vi "Choreo_Util_ConvertTrajectoryToRelative.vi"(11 "ChoreoTrajectory":T1) -> (3 "Flipped Trajectory":T1)   [LabVIEW 2019]
doc: "trajectory, mirrored across the field midline.\n\nInputs: \n - ChoreoTrajectory - cluster - Input trajectory\n\nOutputs:\n - Flipped Trajectory - cluster - trajectory, mirrored across the field midline."
uses:
  TypeDef/ChoreoTrajectory.ctl
  TypeDef/ChoreoTrajectoryState.ctl
  Choreo_TrajectoryState_New.vi
  Choreo_TrajectoryState_GetAll.vi
  Choreo_TrajectoryState_FieldWidth.vi
  ChoreoLib.lvlib
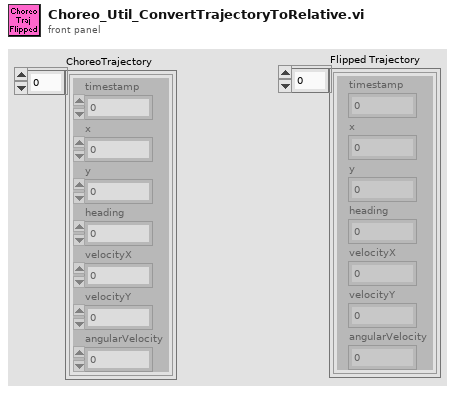
[diagram p1: front panel]
types:
  T1 = typedef "ChoreoLib.lvlib/ChoreoTrajectory.ctl" = T2[]
  T2 = typedef "ChoreoLib.lvlib/ChoreoTrajectoryState.ctl" = cluster{"timestamp":dbl, "x":dbl, "y":dbl, "heading":dbl, "velocityX":dbl, "velocityY":dbl, "angularVelocity":dbl}
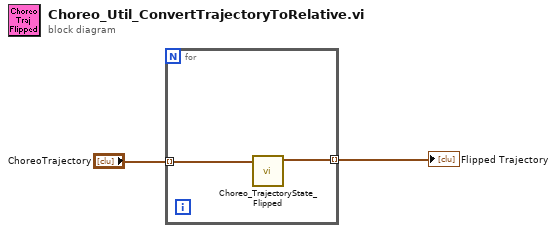
[diagram p0: block diagram]
diagram:
  n1 = for {
    tunnel: "ChoreoTrajectory" -> [w4] mode=indexing
    tunnel: [w3] -> w1 mode=indexing
    n2 = call "Choreo_TrajectoryState_Flipped.vi"("ChoreoTrajectoryState"=w4) -> ("flipped ChoreoTrajectoryState"=w3:T2)  [unwired: 10 in]
  }
  "Flipped Trajectory" <- w1
